vi "search for available lvclass files.vi"(8 "error in":errorcluster, 10 "Folders to Exclude":string[](array[string]), 11 "Plugin Search Paths":path[](array[path])) -> (0 "error out":errorcluster, 3 "discovered classes":path[](array[path]))   [LabVIEW 2025, in "CEF.lvlib"]
doc: "Finds all lvclass files, even inside llb and lvlibp files. Removes any in a folder titled \"\\builds\\\".Copyright 2017 National Instruments Corporation\n\nLicensed under the Apache License, Version 2.0 (the \"License\"); you may not use this file except in compliance with the License. You may obtain a copy of the License at http://www.apache.org/licenses/LICENSE-2.0\nUnless required by applicable law or agreed to in writing, software distributed under the License is distributed on an \"AS IS\" BASIS, WITHOUT WARRANTIES OR CONDITIONS OF ANY KIND, either express or implied. See the License for the specific language governing permissions and limitations under the License."
uses:
  CEF.lvlib
  <vilib>/Utility/LVLibp/NI_PackedLibraryUtility.lvlib
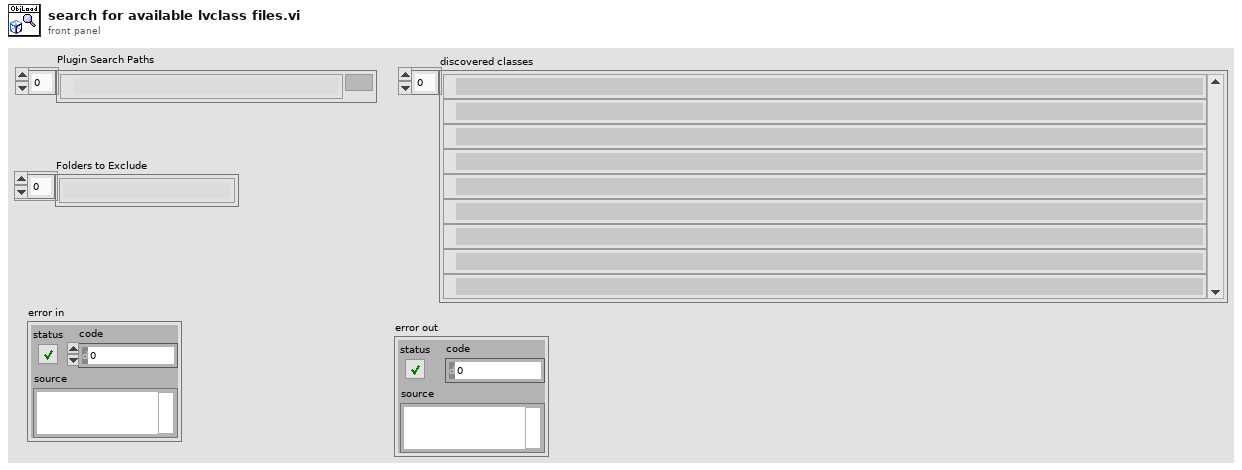
[diagram p1: front panel]
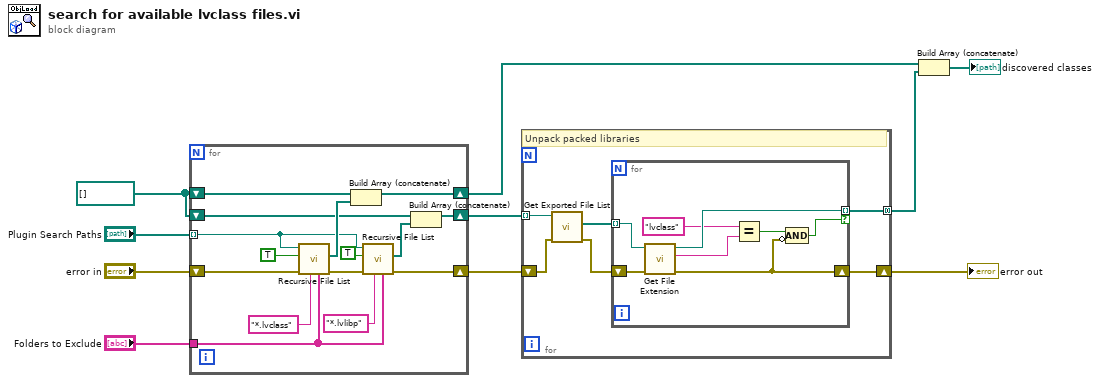
[diagram p0: block diagram]
diagram:
  w5 = path[] [] ("All Files in Dir")
  n1 = for {
    tunnel: "Folders to Exclude" -> [w25]
    shift-right: [w15] -> w7
    shift-left: w5 -> [w16]
    shift-right: [w12] -> w9
    shift-left: w5 -> [w14]
    shift-right: [w19] -> w2
    shift-left: "error in" -> [w18]
    tunnel: "Plugin Search Paths" -> [w11] mode=indexing
    n2 = call <vilib>:"Recursive File List.vi"("Folders to Exclude"=w25, "pattern"="*.lvclass", "error in (no error)"=w18, "Treat LLBs as Folders?"=TRUE, "Folder Path"=w11) -> ("error out"=w22:errorcluster, "All Files in Dir"=w17:path[])  [unwired: 2 in, 3 out]
    n3 = Build Array (concatenate)(w16, w17) -> (w15:path[])
    n4 = call <vilib>:"Recursive File List.vi"("Folders to Exclude"=w25, "pattern"="*.lvlibp", "error in (no error)"=w22, "Treat LLBs as Folders?"=TRUE, "Folder Path"=w11) -> ("error out"=w19:errorcluster, "All Files in Dir"=w13:path[])  [unwired: 2 in, 3 out]
    n5 = Build Array (concatenate)(w14, w13) -> (w12:path[])
  }
  n6 = for {
    tunnel: w9 -> [w31] mode=indexing
    tunnel: [w29] -> w10 mode=concatenating
    shift-right: [w27] -> w1
    shift-left: w2 -> [w28]
    # "Unpack packed libraries"
    n7 = call <vilib>:"Get Exported File List.vi"("error in (no error)"=w28, "packed library path"=w31) -> ("error out"=w26:errorcluster, "paths"=w30:path[])  [unwired: 7 in, 1 out]
    n8 = for {
      tunnel: w30 -> [w39] mode=indexing
      tunnel: [w37] -> w29 mode=indexing if=w36
      shift-right: [w35] -> w27
      shift-left: w26 -> [w34]
      n9 = call <vilib>:"Get File Extension.vi"("error in (no error)"=w34, "file"=w39) -> ("error out"=w35:errorcluster, "lowercase file extension"=w33:string, "dup file"=w37:path)  [unwired: 5 in, 2 out]
      n10 = Equal?(x="lvclass", y=w33) -> (x = y?=w38:bool)
      n11 = Compound Arithmetic op=AND(w38, invert w35) -> (w36:bool)
    }
  }
  "error out" <- w1
  n12 = Build Array (concatenate)(w7, w10) -> (→"discovered classes":path[])
